vi "GetXMLValue.vi"(11 "Path":path) -> (3 "Value":dbl format="%#_13g")   [LabVIEW 2017]
uses:
  <vilib>/Utility/xml.llb/Read From XML File(string).vi
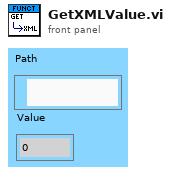
[diagram p1: front panel]
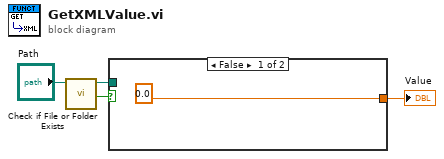
[diagram p0: block diagram]
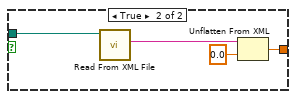
[diagram p2: hidden frame]
diagram:
  n1 = call <vilib>:"Check if File or Folder Exists.vi"("path"="Path") -> ("file or folder exists?"=w3:bool, "dup path"=w2:path)  [unwired: 8 in, 1 out]
  n2 = case shown="False" w3 {
    tunnel: w2 -> [_ w9]
    tunnel: [0.0 w6] -> w1
    frame False {
    }
    frame True {
      n3 = call-poly <vilib>:"Read From XML File.vi"("XML File Path"=w9) -> ("XML Elements"=w8:string)  [unwired: 8 in, 2 out]
      n4 = Unflatten From XML(xml string=w8, type=0.0) -> (value=w6:dbl)  [unwired: 1 in, 1 out]
    }
  }
  "Value" <- w1
